vi "USRP oneTx one Rx_USRP2.vi"() -> ()   [LabVIEW 2021]
uses:
  <vilib>/addons/Modulation/Analog/controls/Complex Data Waveform.ctl
  <vilib>/measure/maspectr.llb/Power Spectrum and PSD Export Mode.ctl
  system stop.vi
  <vilib>/measure/matone.llb/Extract Single Tone Information 1 Chan (CDB).vi
  <vilib>/measure/maspectr.llb/FFT Power Spectrum and PSD for 1 Chan (CDB).vi
  <instrlib>/niUSRP/niUSRP Fetch Rx Data (CDB Cluster).vi
  <instrlib>/niUSRP/niUSRP Write Tx Data (CDB Cluster).vi
  <vilib>/addons/Modulation/niAMT.lvlib
  <vilib>/measure/NI_MAPro.lvlib
panel:
  in  "Tab Control":T1(tab)
  in  "IQ rate Tx":dbl=100000.0 format="%#_6p"
  in  "carrier frequency Tx":dbl=100000.0 format="%#_6p"
  in  "Tx Gain":dbl format="%#_6f"
  in  "Tx IP":refnum<k15>
  out "coerced IQ rate Tx":dbl=100000.0 format="%#_6p"
  out "coerced carrier frequency Tx":dbl=100000.0 format="%#_6p"
  in  "Rx IP":refnum<k15>
  in  "Rx gain":dbl format="%#_6f"
  in  "Frequency":dbl format="%#_13g"
  in  "Duration":dbl format="%#_13g"
  out "coerced IQ rate Rx":dbl=100000.0 format="%#_6p"
  out "coerced carrier frequency Rx":dbl=100000.0 format="%#_6p"
  in  "number of samples":i64=100000
  out "Waveform Graph":dbl[](graph)
  out "Received Waveform Graph":cluster{"f0":dbl, "df":dbl, "magnitude":dbl[]}(graph)
  out "detected frequency":dbl format="%.2p"
  out "detected Amplitude in dBm":dbl format="%.2p"
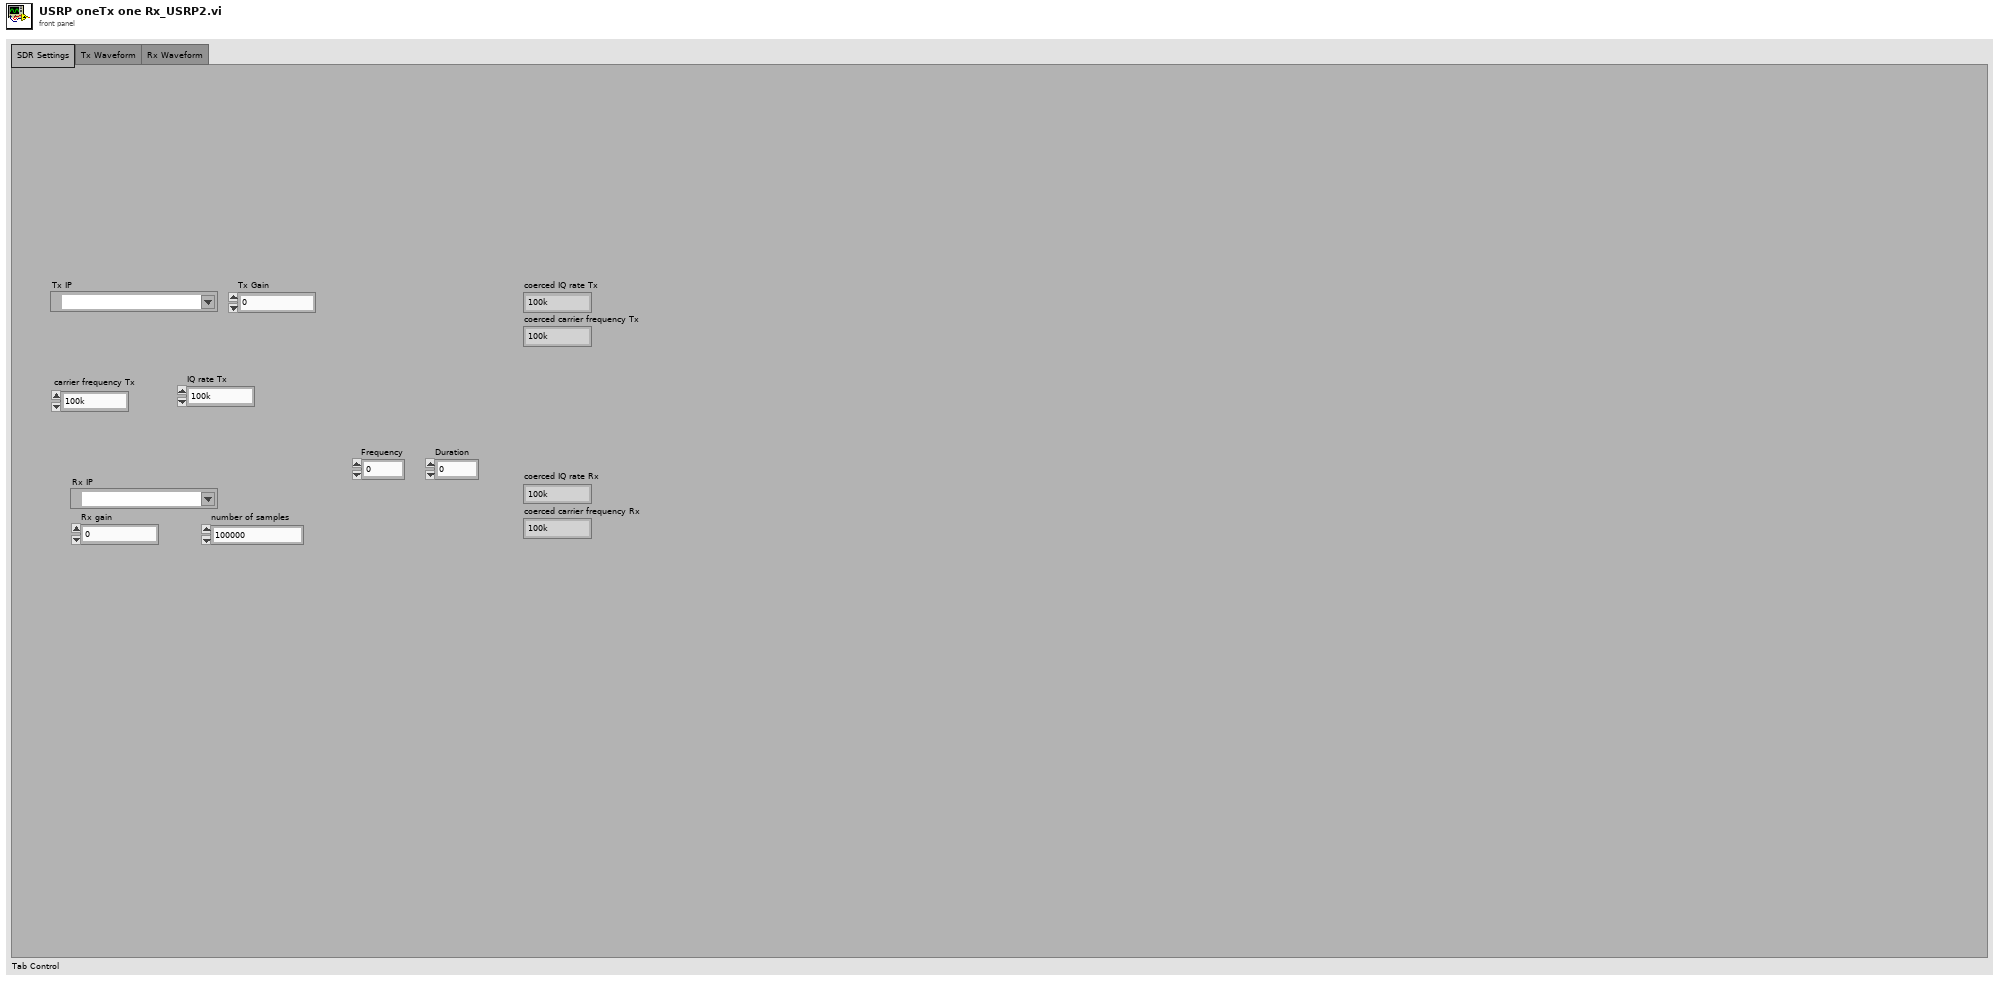
[diagram p1: front panel]
types:
  T1 = enum32{"SDR Settings", "Tx Waveform", "Rx Waveform"}
  T2 = typedef "niAMT.lvlib/Complex Data Waveform.ctl" = cluster{"t0":dbl, "dt":dbl, "Y":cdb[]}
  T3 = typedef "NI_MAPro.lvlib/Power Spectrum and PSD Export Mode.ctl" = u16
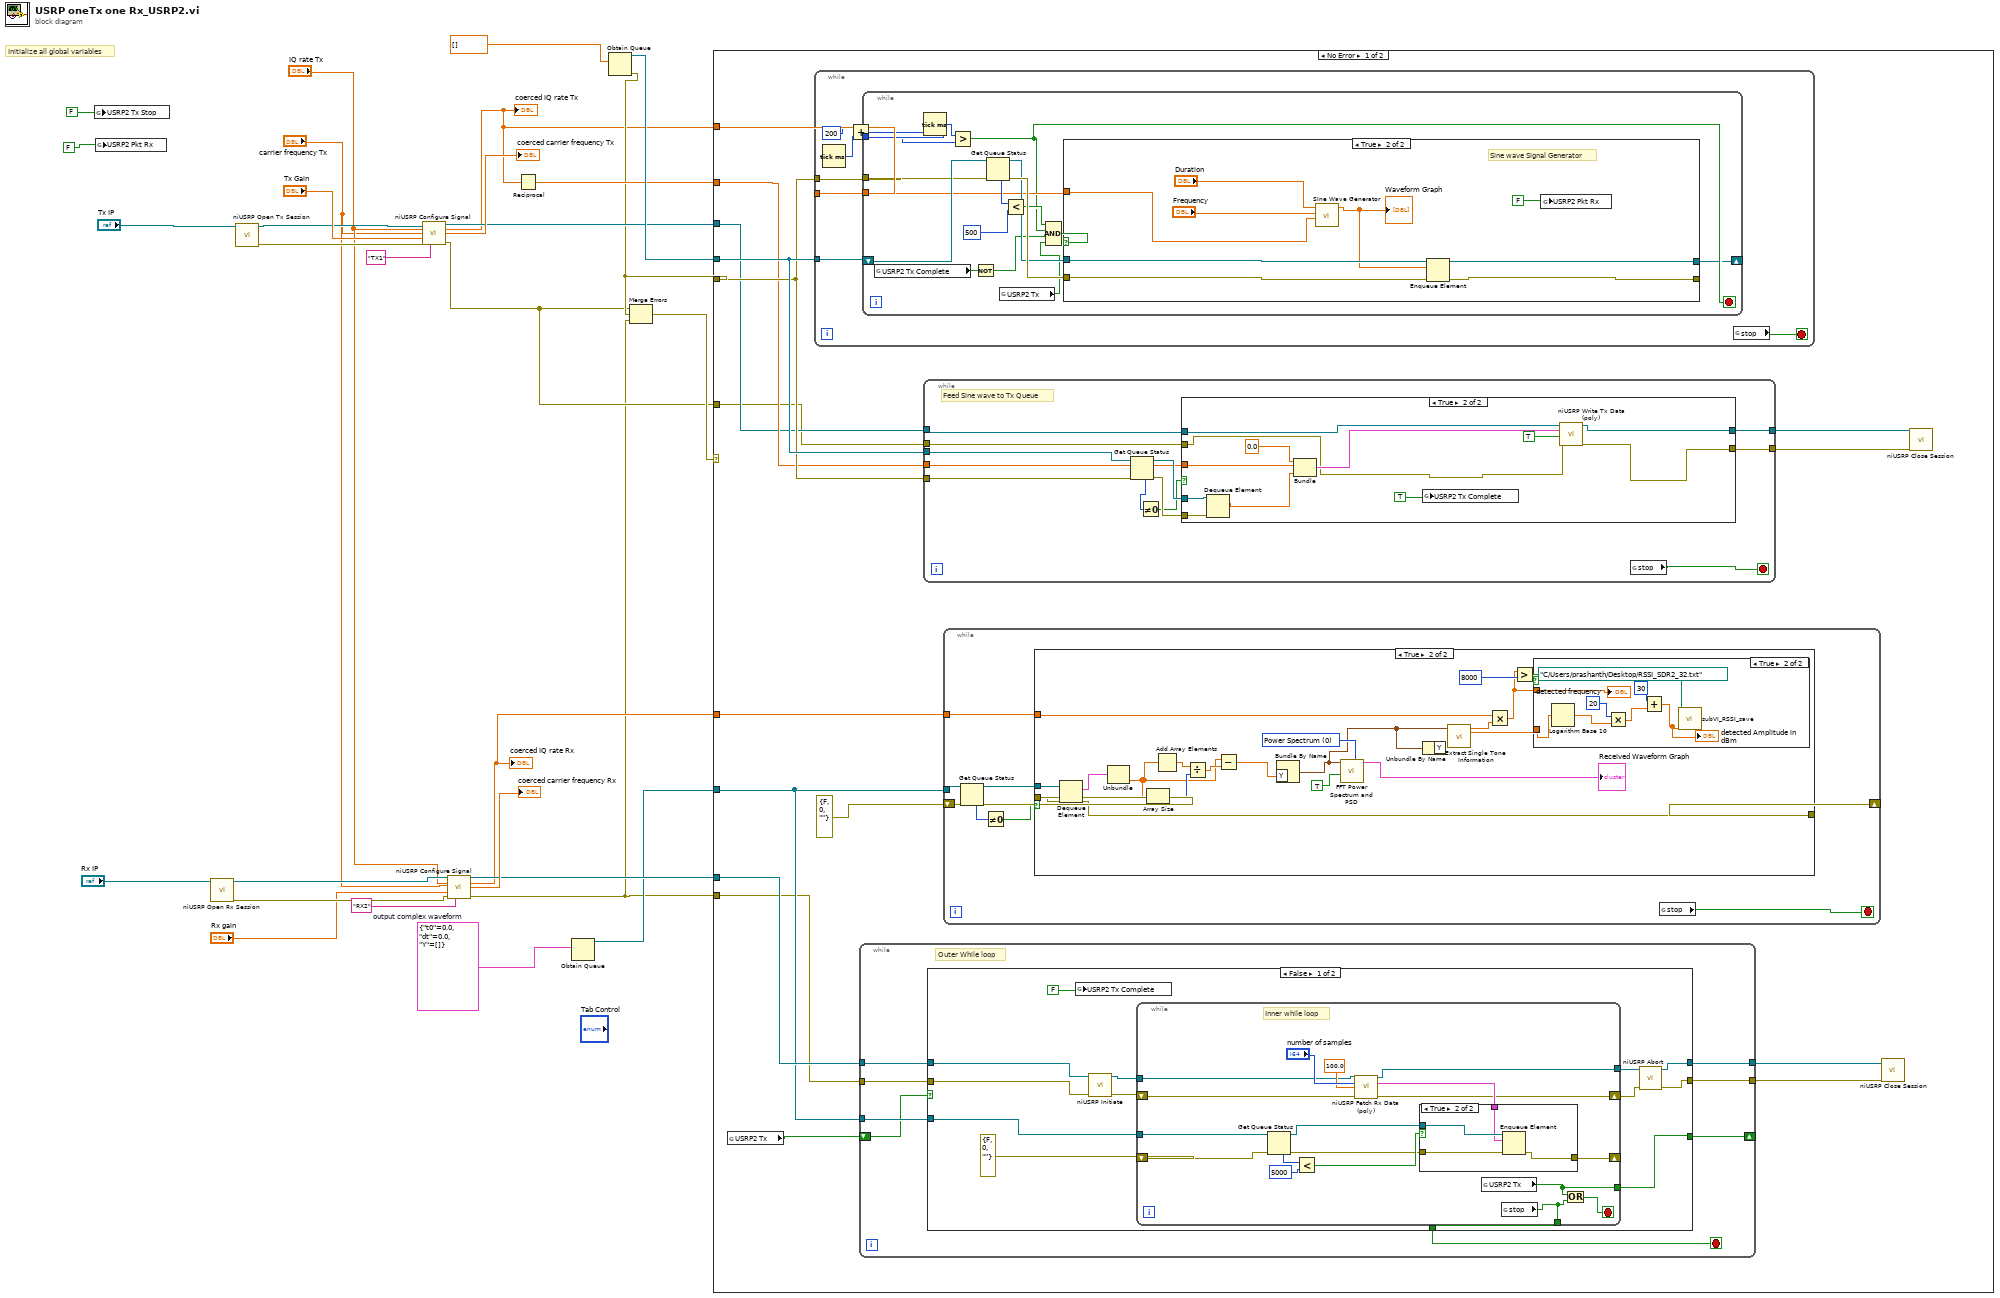
[diagram p0: block diagram]
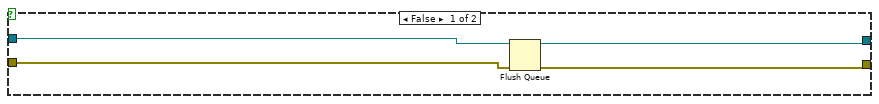
[diagram p2: hidden frame]
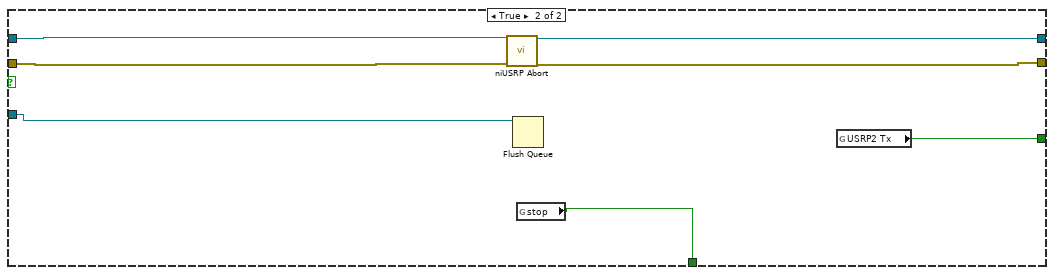
[diagram p4: hidden frame]
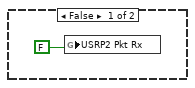
[diagram p6: hidden frame]
diagram:
  w6 = T2 {"t0"=0.0, "dt"=0.0, "Y"=[]}  # output complex waveform
  # "Initialize all global variables"
  n1 = global write "system stop.vi" "USRP2 Tx Stop"(FALSE) -> ()
  n2 = global write "system stop.vi" "USRP2 Pkt Rx"(FALSE) -> ()
  n3 = call <instrlib>:"niUSRP Open Rx Session.vi"("device names"="Rx IP") -> ("session handle out"=w13:refnum<k15>, "error out"=w12:errorcluster)  [unwired: 13 in]
  n4 = call <instrlib>:"niUSRP Open Tx Session.vi"("device names"="Tx IP") -> ("session handle out"=w27:refnum<k15>, "error out"=w26:errorcluster)  [unwired: 13 in]
  n5 = call <instrlib>:"niUSRP Configure Signal.vi"("session handle"=w27, "IQ rate"="IQ rate Tx", "carrier frequency"="carrier frequency Tx", "gain"="Tx Gain", "error in (no error)"=w26, "active antenna"="TX1") -> ("session handle out"=w20:refnum<k15>, "coerced IQ rate"=w17:dbl, "coerced carrier frequency"=→"coerced carrier frequency Tx":dbl, "error out"=w16:errorcluster)  [unwired: 5 in, 1 out]
  "coerced IQ rate Tx" <- w17
  n6 = call <instrlib>:"niUSRP Configure Signal.vi"("session handle"=w13, "IQ rate"="IQ rate Tx", "carrier frequency"="carrier frequency Tx", "gain"="Rx gain", "error in (no error)"=w12, "active antenna"="RX2") -> ("session handle out"=w7:refnum<k15>, "coerced IQ rate"=w4:dbl, "coerced carrier frequency"=→"coerced carrier frequency Rx":dbl, "error out"=w2:errorcluster)  [unwired: 5 in, 1 out]
  "coerced IQ rate Rx" <- w4
  n7 = Reciprocal(x=w17) -> (1/x=w19:dbl)
  n8 = Obtain Queue(element data type=w6) -> (queue out=w5:refnum<queue>)  [unwired: 4 in, 2 out]
  n9 = Obtain Queue(element data type=dbl[] []) -> (queue out=w21:refnum<queue>, error out=w18:errorcluster)  [unwired: 4 in, 1 out]
  n10 = Merge Errors(w16, w18, w2) -> (w23:errorcluster)
  n11 = case shown="No Error" w23 {
    tunnel: w18 -> [w44 _]
    tunnel: w21 -> [w45 _]
    tunnel: w20 -> [w42 _]
    tunnel: w19 -> [w43 _]
    tunnel: w17 -> [w41 _]
    tunnel: w16 -> [w40 _]
    tunnel: w7 -> [w38 _]
    tunnel: w5 -> [w37 _]
    tunnel: w4 -> [w36 _]
    tunnel: w2 -> [w35 _]
    frame No Error {
      n12 = global read "system stop.vi" "USRP2 Tx"() -> (w30:bool)
      n13 = while {
        tunnel: w45 -> [w52]
        tunnel: w44 -> [w51]
        tunnel: w41 -> [w50]
        stop <- w49 stop-if-true
        n14 = Tick Count (ms)() -> (millisecond timer value=w48:u32)
        n15 = Add(x=200, y=w48) -> (x+y=w47:u32)
        n16 = while {
          tunnel: w51 -> [w63]
          tunnel: w50 -> [w62]
          tunnel: w47 -> [w57]
          shift-right: [w53] -> _
          shift-left: w52 -> [w64]
          stop <- w56 stop-if-true
          n17 = global read "system stop.vi" "USRP2 Tx Complete"() -> (w55:bool)
          n18 = Tick Count (ms)() -> (millisecond timer value=w58:u32)
          n19 = Greater?(x=w58, y=w57) -> (0:w56:bool)
          n20 = Not(x=w55) -> (.not. x?=w54:bool)
          n21 = Get Queue Status(queue=w64, error in (no error)=w63) -> (queue out=w65:refnum<queue>, error out=w66:errorcluster, # elements in queue=w68:i32)  [unwired: 1 in, 5 out]
          n22 = global read "system stop.vi" "USRP2 Tx"() -> (w60:bool)
          n23 = Less?(x=w68, y=500) -> (x < y?=w61:bool)
          n24 = Compound Arithmetic op=AND(w61, w56, w54, w60) -> (w59:bool)
          n25 = case shown="True" w59 {
            tunnel: w66 -> [w71 w81]
            tunnel: w65 -> [w72 w80]
            tunnel: [w70 w79] -> w53
            tunnel: [w69 w78] -> _
            tunnel: w62 -> [_ w75]
            frame False {
              n26 = Flush Queue(queue=w72, error in (no error)=w71) -> (queue out=w70:refnum<queue>, error out=w69:errorcluster)  [unwired: 1 out]
            }
            frame True {
              # "Sine wave Signal Generator"
              n27 = call "SIne Wave Generator.vi"("Sampling rate"=w75, "Frequency"="Frequency", "Duration"="Duration") -> ("Array"=w74:dbl[])  [unwired: 7 in, 1 out]
              "Waveform Graph" <- w74
              n28 = Enqueue Element(queue=w80, element=w74, error in (no error)=w81) -> (queue out=w79:refnum<queue>, error out=w78:errorcluster)  [unwired: 1 in, 1 out]
              n29 = global write "system stop.vi" "USRP2 Pkt Rx"(FALSE) -> ()
            }
          }
        }
        n30 = global read "system stop.vi" "stop"() -> (w49:bool)
      }
      n31 = while {
        tunnel: w38 -> [w89]
        tunnel: w37 -> [w88]
        tunnel: w35 -> [w86]
        tunnel: [w85] -> w32
        tunnel: [w84] -> w31
        shift-right: [w82] -> _
        shift-left: w30 -> [w83]
        stop <- w87 stop-if-true
        # "Outer While loop"
        n32 = case shown="False" w83 {
          tunnel: w89 -> [w97 w130]
          tunnel: w88 -> [w102 w126]
          tunnel: [w100 w132] -> w87
          tunnel: w86 -> [w95 w128]
          tunnel: [w92 w129] -> w85
          tunnel: [w91 w127] -> w84
          tunnel: [w99 w131] -> w82
          frame False {
            n33 = global write "system stop.vi" "USRP2 Tx Complete"(FALSE) -> ()
            n34 = call <instrlib>:"niUSRP Initiate.vi"("session handle"=w97, "error in (no error)"=w95) -> ("session handle out"=w96:refnum<k15>, "error out"=w94:errorcluster)  [unwired: 12 in]
            n35 = while {
              tunnel: w102 -> [w120]
              shift-right: [w103] -> w90
              shift-left: w94 -> [w119]
              shift-right: [w118] -> _
              shift-left: errorcluster {"status"=FALSE, "code"=0, "source"=""} ("error in (no error)") -> [w117]
              tunnel: [w108] -> w100
              tunnel: [w107] -> w99
              tunnel: w96 -> [w105]
              tunnel: [w104] -> w93
              stop <- w109 stop-if-true
              # "Inner while loop"
              n36 = Get Queue Status(queue=w120, error in (no error)=w117) -> (queue out=w112:refnum<queue>, error out=w113:errorcluster, # elements in queue=w116:i32)  [unwired: 1 in, 5 out]
              n37 = Less?(x=w116, y=5000) -> (x < y?=w114:bool)
              n38 = call-poly <instrlib>:"niUSRP Fetch Rx Data (poly).vi"("session handle"=w105, "number of samples"="number of samples", "timeout"=100.0, "error in (no error)"=w119) -> ("session handle out"=w104:refnum<k15>, "data"=w110:cluster{"t0":dbl, "dt":dbl, "Y":cdb[]}, "error out"=w103:errorcluster)  [unwired: 8 in, 1 out]
              n39 = case shown="True" w114 {
                tunnel: w113 -> [w121 w125]
                tunnel: w112 -> [_ w124]
                tunnel: w110 -> [_ w123]
                tunnel: [w121 w122] -> w118
                frame False {
                }
                frame True {
                  n40 = Enqueue Element(queue=w124, element=w123, error in (no error)=w125) -> (error out=w122:errorcluster)  [unwired: 1 in, 2 out]
                }
              }
              n41 = global read "system stop.vi" "USRP2 Tx"() -> (w107:bool)
              n42 = global read "system stop.vi" "stop"() -> (w108:bool)
              n43 = Or(x=w107, y=w108) -> (x .or. y?=w109:bool)
            }
            n44 = call <instrlib>:"niUSRP Abort.vi"("session handle"=w93, "error in (no error)"=w90) -> ("session handle out"=w92:refnum<k15>, "error out"=w91:errorcluster)  [unwired: 12 in]
          }
          frame True {
            n45 = call <instrlib>:"niUSRP Abort.vi"("session handle"=w130, "error in (no error)"=w128) -> ("session handle out"=w129:refnum<k15>, "error out"=w127:errorcluster)  [unwired: 12 in]
            n46 = Flush Queue(queue=w126) -> ()  [unwired: 1 in, 3 out]
            n47 = global read "system stop.vi" "stop"() -> (w132:bool)
            n48 = global read "system stop.vi" "USRP2 Tx"() -> (w131:bool)
          }
        }
      }
      n49 = while {
        tunnel: w45 -> [w182]
        tunnel: w44 -> [w179]
        tunnel: w43 -> [w178]
        tunnel: w42 -> [w176]
        tunnel: w40 -> [w174]
        tunnel: [w172] -> w34
        tunnel: [w171] -> w33
        stop <- w173 stop-if-true
        # "Feed Sine wave to Tx Queue"
        n50 = Get Queue Status(queue=w182, error in (no error)=w179) -> (queue out=w181:refnum<queue>, error out=w180:errorcluster, # elements in queue=w177:i32)  [unwired: 1 in, 5 out]
        n51 = Not Equal To 0?(x=w177) -> (x != 0?=w175:bool)
        n52 = case shown="True" w175 {
          tunnel: w181 -> [_ w196]
          tunnel: w180 -> [_ w195]
          tunnel: w178 -> [_ w194]
          tunnel: w176 -> [w184 w192]
          tunnel: w174 -> [w183 w186]
          tunnel: [w184 w188] -> w172
          tunnel: [w183 w185] -> w171
          frame False {
          }
          frame True {
            n53 = Dequeue Element(queue=w196, error in (no error)=w195) -> (element=w191:dbl[])  [unwired: 1 in, 3 out]
            n54 = Bundle(0.0, w194, w191) -> (w193:cluster{dbl, dbl, dbl[]})  [unwired: 1 in]
            n55 = global write "system stop.vi" "USRP2 Tx Complete"(TRUE) -> ()
            n56 = call-poly <instrlib>:"niUSRP Write Tx Data (poly).vi"("session handle"=w192, "data"=w193, "end of data?"=TRUE, "error in (no error)"=w186) -> ("session handle out"=w188:refnum<k15>, "error out"=w185:errorcluster)  [unwired: 10 in]
          }
        }
        n57 = global read "system stop.vi" "stop"() -> (w173:bool)
      }
      n58 = while {
        tunnel: w37 -> [w138]
        shift-right: [w135] -> _
        shift-left: errorcluster {"status"=FALSE, "code"=0, "source"=""} ("error in (no error)") -> [w137]
        tunnel: w36 -> [w134]
        stop <- w133 stop-if-true
        n59 = Get Queue Status(queue=w138, error in (no error)=w137) -> (queue out=w140:refnum<queue>, error out=w139:errorcluster, # elements in queue=w141:i32)  [unwired: 1 in, 5 out]
        n60 = Not Equal To 0?(x=w141) -> (x != 0?=w136:bool)
        n61 = case shown="True" w136 {
          tunnel: w140 -> [_ w161]
          tunnel: w139 -> [w142 w155]
          tunnel: [w142 w153] -> w135
          tunnel: w134 -> [_ w152]
          frame False {
          }
          frame True {
            w158 = T3 0 items=["Power Spectrum", "Power Spectral Density"] ("export mode")
            n62 = Dequeue Element(queue=w161, error in (no error)=w155) -> (element=w154:T2, error out=w153:errorcluster)  [unwired: 1 in, 2 out]
            n63 = Unbundle(w154) -> ("Y"=w144:cdb[])  [unwired: 2 out]
            n64 = Array Size(array=w144) -> (size(s)=w146:i32)
            n65 = Add Array Elements(numeric array=w144) -> (sum=w147:cdb)
            n66 = Divide(x=w147, y=w146) -> (x/y=w145:cdb)
            n67 = Subtract(x=w144, y=w145) -> (x-y=w143:cdb[])
            n68 = Bundle By Name("Y"=w143) -> (w156:waveform(cdb))  [unwired: 1 in]
            n69 = call-poly <vilib>:"FFT Power Spectrum and PSD.vi"("export mode"=w158, "dB On (F)"=TRUE, "time signal"=w156) -> ("Power Spectrum / PSD"=→"Received Waveform Graph":cluster{"f0":dbl, "df":dbl, "magnitude":dbl[]})  [unwired: 5 in, 3 out]
            n70 = Unbundle By Name(w156) -> ()  [unwired: 1 out]
            n71 = call-poly <vilib>:"Extract Single Tone Information.vi"("time signal in"=w156) -> ("detected amplitude"=w148:dbl, "detected frequency"=w157:dbl)  [unwired: 5 in, 4 out]
            n72 = Multiply(x=w152, y=w157) -> (x*y=w149:dbl)
            n73 = Greater?(x=w149, y=8000) -> (0:w150:bool)
            n74 = case shown="True" w150 {
              tunnel: w149 -> [_ w170]
              tunnel: w148 -> [_ w169]
              frame False {
                n75 = global write "system stop.vi" "USRP2 Pkt Rx"(FALSE) -> ()
              }
              frame True {
                n76 = Logarithm Base 10(1:w169) -> (0:w167:dbl)
                n77 = Multiply(x=20, y=w167) -> (x*y=w164:dbl)
                n78 = Add(x=30, y=w164) -> (x+y=w163:dbl)
                "detected Amplitude in dBm" <- w163
                n79 = call "subVI_RSSI_save.vi"("RSSI"=w163, "file path (dialog if empty)"=path "C:/Users/prashanth/Desktop/RSSI_SDR2_32.txt") -> ()  [unwired: 10 in]
                "detected frequency" <- w170
              }
            }
          }
        }
        n80 = global read "system stop.vi" "stop"() -> (w133:bool)
      }
      n81 = call <instrlib>:"niUSRP Close Session.vi"("session handle"=w32, "error in (no error)"=w31) -> ()  [unwired: 13 in, 1 out]
      n82 = call <instrlib>:"niUSRP Close Session.vi"("session handle"=w34, "error in (no error)"=w33) -> ()  [unwired: 13 in, 1 out]
    }
    frame Error {
    }
  }
